vi "ProcessData.vi"(8 "error in (no error)":errorcluster, 10 "Analog Data":T2, 11 "TrialBasedExperiment in":refnum<class "MatlabExperiment.lvclass">) -> (0 "error out":errorcluster, 1 "Fixated":bool, 2 "Trigger":T1=enum."Broke Fixation", 3 "TrialBasedExperiment out":refnum<class "MatlabExperiment.lvclass">)   [LabVIEW 2010]
uses:
  Trial Based Experiment.lvsc/Trigger.ctl
  Trial Based Experiment.lvsc
  Core SubVIs/Core SubVIs.lvlib
  <vilib>/measure/NI_MAPro.lvlib
  <vilib>/measure/madcrms.llb/Basic Averaged DC-RMS for 1 Chan.vi
  MatlabExperiment.lvclass
  Core SubVIs/Controls/TYPE - Analog Data.ctl
panel:
  in  "Toggle":bool
  in  "Radius":dbl
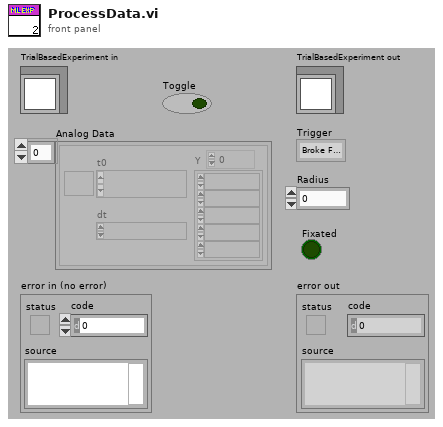
[diagram p1: front panel]
types:
  T1 = typedef "Trial Based Experiment.lvsc/Trigger.ctl" = enum16{"NULL", "Fixated", "Broke Fixation", "Stop", "Correct Response", "Incorrect Response", "Timeout"}
  T2 = typedef "Core SubVIs.lvlib/TYPE - Analog Data.ctl" = waveform(dbl)[]
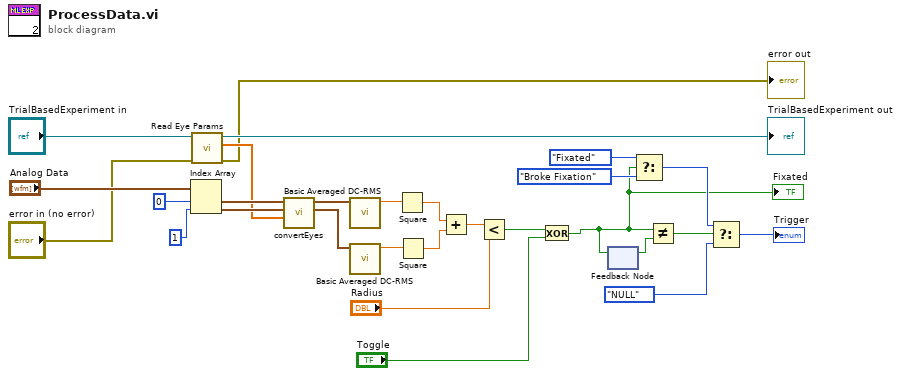
[diagram p0: block diagram]
diagram:
  n1 = Index Array(array="Analog Data", index #1=0 ("index"), index #2=1 ("index")) -> (element #1=w25:waveform(dbl), element #2=w24:waveform(dbl))
  n2 = call-dynamic "Read Eye Params.vi"("error in (no error)"="error in (no error)", "TrialBasedExperiment in"="TrialBasedExperiment in") -> ("error out"=→"error out":errorcluster, "Eye Params"=w6:dbl[], "TrialBasedExperiment out"=→"TrialBasedExperiment out":refnum<class "MatlabExperiment.lvclass">)  [unwired: 7 in]
  n3 = call "convertEyes.vi"("Params"=w6, "Vertical"=w24, "Horizontal"=w25) -> ("Vertical Calibrated"=w22:waveform(dbl), "Horizontal Calibrated"=w23:waveform(dbl))  [unwired: 7 in]
  n4 = call-poly <vilib>:"Basic Averaged DC-RMS.vi"("signal in"=w23) -> ("DC value"=w21:dbl)  [unwired: 7 in, 3 out]
  n5 = call-poly <vilib>:"Basic Averaged DC-RMS.vi"("signal in"=w22) -> ("DC value"=w20:dbl)  [unwired: 7 in, 3 out]
  n6 = Square(x=w21) -> (x^2=w19:dbl)
  n7 = Square(x=w20) -> (x^2=w18:dbl)
  n8 = Add(x=w19, y=w18) -> (x+y=w17:dbl)
  n9 = Less?(x=w17, y="Radius") -> (x < y?=w2:bool)
  n10 = Exclusive Or(1:"Toggle", 2:w2) -> (0:w1:bool)
  "Fixated" <- w1
  n11 = feedback #1() -> (w15:bool)  [unwired: 1 in]
  n12 = feedback-in #1(w1) -> ()
  n13 = Select(t=Trigger."Fixated" ("Trigger"), s=w1, f=Trigger."Broke Fixation" ("Trigger")) -> (s? t:f=w12:T1)
  n14 = Not Equal?(x=w1, y=w15) -> (x != y?=w14:bool)
  n15 = Select(t=w12, s=w14, f=Trigger."NULL" ("Trigger")) -> (s? t:f=→"Trigger":T1)
